vi "PS Control.vi"() -> ()   [LabVIEW 2023]
doc: "Author: Scott Hannahs <sth@magnet.fsu.edu>\nCopyright 2018 Florida State University, All rights reserved."
uses:
  SCM4 Interlock/RT SubVIs/RT System Auth Level.ctl
  SCM4 Interlock/RT SubVIs/PS Action Control.ctl
  <vilib>/Utility/miscctls.llb/LVOffsetAndMultiplierTypeDef.ctl
  SCM4 Interlock/RT SubVIs/Interlock RT FPGA Status Info.ctl
  SCM4 Interlock/FPGA SubVIs/FPGA Crowbar State.ctl
  SCM4 Interlock/RT SubVIs/Switch Box Status.ctl
  SubVIs/Interlock 32T Net Client Globals.vi
  TCP Functions/TCP Read Length and Value (STR).vi
  <vilib>/Utility/miscctls.llb/LVRectTypeDef.ctl
  <vilib>/Utility/miscctls.llb/LVPointTypeDef.ctl
panel:
  in  "Clear Quench":bool
  out "# Clients":u32
  out "Currents":dbl[][](graph)
  in  "Client Loop Time (mS)":u32=100
  out "Start DateStamp":timestamp format="%<%H:%M:%S%4u\n%Y/%m/%d>T"
  out "Version RT System":string
  out "Version FPGA":string
  in  "Password":string
  out "Authorized":T1
  in  "Slew Rate [T/min]":dbl format="%.3g"
  out "Field [T]":dbl format="%.5f"
  in  "Setpoint [T]":dbl format="%.6g"
  in  "PS Action":T2=enum."Hold"
  out "Version":string
  in  "stop":bool
  # "NHMFL 32T User Control"
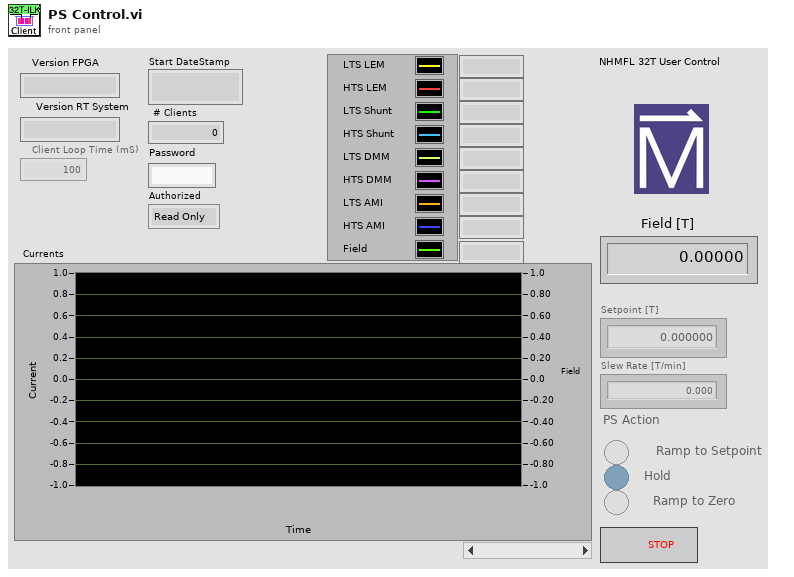
[diagram p1: front panel]
types:
  T1 = typedef "RT System Auth Level.ctl" = enum16{"Read Only", "User", "Operator", "Admin"}
  T2 = typedef "PS Action Control.ctl" = enum32{"Ramp to Setpoint", "Hold", "Ramp to Zero"}
  T3 = enum8{"Enabled", "Disabled", "Disabled and Grayed Out"}
  T4 = typedef "LVPointTypeDef.ctl" = cluster{"Horizontal":i16, "Vertical":i16}
  T5 = typedef "LVRectTypeDef.ctl" = cluster{"Left":i16, "Top":i16, "Right":i16, "Bottom":i16}
  T6 = typedef "LVOffsetAndMultiplierTypeDef.ctl" = cluster{"Offset":dbl, "Multiplier":dbl}
  T7 = enum16{"Standard", "Buffered", "CRLF", "Immediate"}
  T8 = typedef "Interlock RT FPGA Status Info.ctl" = cluster{"Authorized":T1, "# Clients":u32, "Chassis Temperature":fxp<+/-,16,14>, "Secondary QD Time Constant":enum16{"2000 mS", "1000 mS", "200 mS", "50 mS"}, "Crowbar Latch State":T9, "Crowbar Reset Countdown Length (ms)":i32, "Crowbar Reset Countdown":i32, "Ramp To Zero Fault":u32, "Crowbar Fault":u16, "Protection Logic V":dbl, "Quench Loop":dbl, "HTS LEM":dbl, "HTS Shunt":dbl, "LTS LEM":dbl, "LTS Shunt":dbl, "Ramp To Zero":bool, "2 Crowbar Reset Key":bool, "7 Crowbar LED":bool, "15 Close Switch Box 2 Contactor":bool, "HTS Voltage":dbl, "LTS Voltage":dbl, "DAQ Loop Ticks":u32, "PQD WDT Loop Tics":u32, "Main Loop Ticks":u32, "PS Check Loop Ticks":u32, "RTZ Loop Ticks":u32, "Watchdog Loop Ticks":u32, "LHe Level 1":dbl, "LHe Level 2":dbl, "HTS DMM":dbl, "LTS DMM":dbl, "HTS AMI430":dbl, "LTS AMI430":dbl, "Battery Monitor Alarm":bool, "Switch Box Status":T10, "PS Action":T2, "Setpoint [T]":dbl, "Field [T]":dbl, "Slew rate [T/min]":dbl, "Recorded error":errorcluster, "Last Batt Comm":timestamp, "Batt Alarm Text":string, "PS Comm Time (ms)":u32, "DMM Comm Time (ms)":u32, "PS Model Cluster":cluster{"HTS B_I0":dbl, "LTS B_I0":dbl, "HTS Bmax":dbl, "LTS Bmax":dbl, "Max combined rate (T/min)":dbl}, "HTS Setpoint [A]":dbl, "HTS Slew [A/S]":dbl, "LTS Setpoint [A]":dbl, "LTS Slew [A/S]":dbl}
  T9 = typedef "FPGA Crowbar State.ctl" = enum16{"Run", "Crowbar", "Reset Countdown"}
  T10 = typedef "Switch Box Status.ctl" = cluster{"Battery Voltage":dbl, "SwBox 1 Contactor V":dbl, "SwBox 2 Contactor V":dbl, "Battery Ground V":dbl}
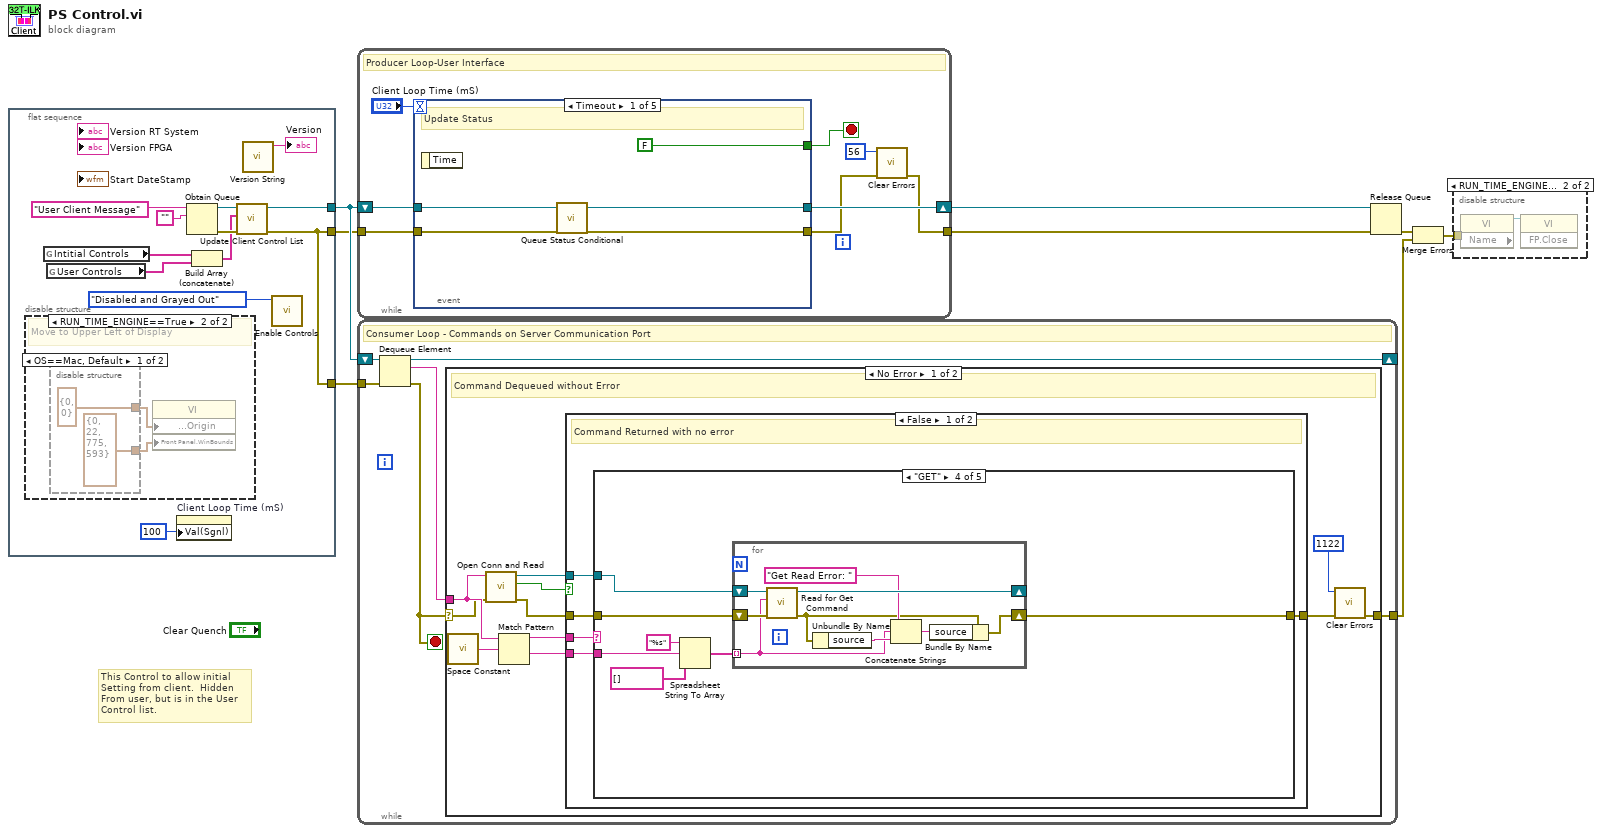
[diagram p0: block diagram]
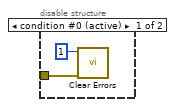
[diagram p2: hidden frame]
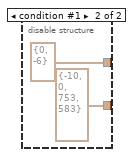
[diagram p4: hidden frame]
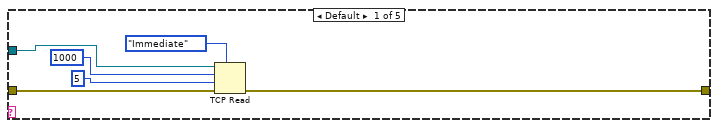
[diagram p5: hidden frame]
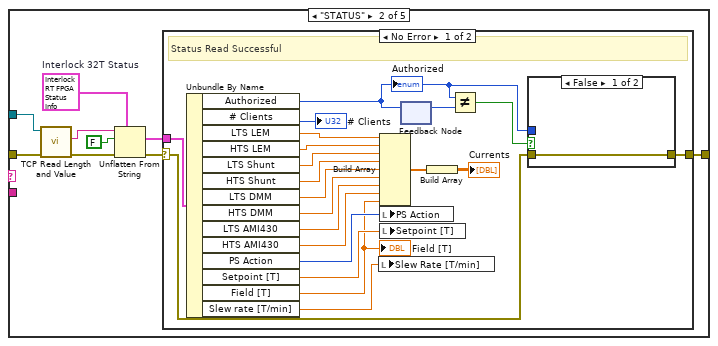
[diagram p6: hidden frame]
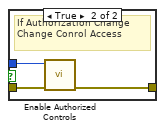
[diagram p7: hidden frame]
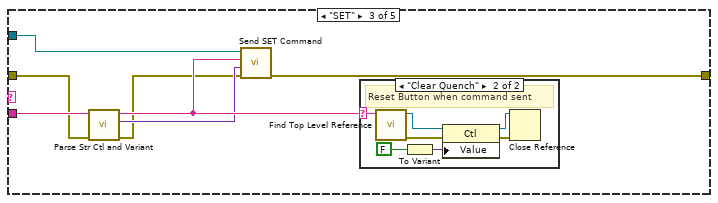
[diagram p9: hidden frame]
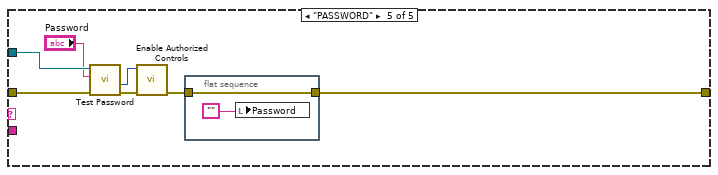
[diagram p11: hidden frame]
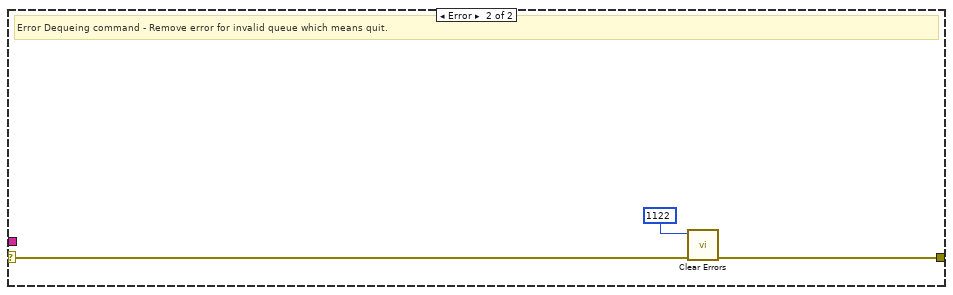
[diagram p13: hidden frame]
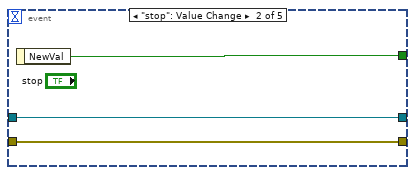
[diagram p14: hidden frame]
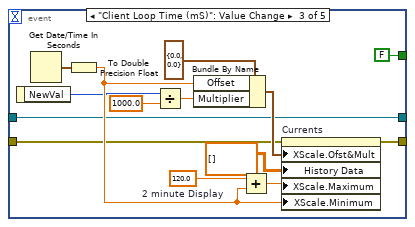
[diagram p15: hidden frame]
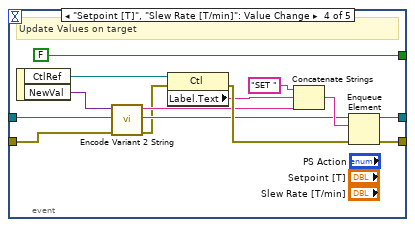
[diagram p16: hidden frame]
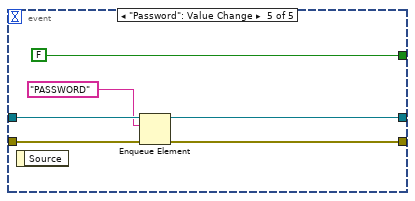
[diagram p17: hidden frame]
diagram:
  # "This Control to allow initial\nSetting from client.  Hidden\nFrom user, but is in the User\nControl list."
  n1 = flat-sequence {
    tunnel: [w20] -> w6
    tunnel: [w10] -> w3
    tunnel: [w10] -> w1
    frame #0 {
      n2 = disable-structure shown="RUN_TIME_ENGINE==True" {
        frame condition #0 (active) {
        }
        frame condition #1 {
          # "Move to Upper Left of Display"
          n3 = disable-structure shown="OS==Mac, Default" {
            disable-tunnel: [T5 {"Left"=0, "Top"=22, "Right"=775, "Bottom"=593} ("Front Panel Window:Window Bounds") T5 {"Left"=-10, "Top"=0, "Right"=753, "Bottom"=583} ("Front Panel Window:Window Bounds")] -> w22
            disable-tunnel: [T4 {"Horizontal"=0, "Vertical"=0} ("Front Panel Window:Origin") T4 {"Horizontal"=0, "Vertical"=-6} ("Front Panel Window:Origin")] -> w21
            frame condition #0 (active) {
            }
            frame condition #1 {
            }
          }
          n4 = property class="VI"("Front Panel Window:Origin"=w21, "Front Panel.WinBounds"=w22) -> ()  [unwired: 2 in, 2 out]
        }
      }
      n5 = global read "Interlock 32T Net Client Globals.vi" "Intitial Controls"() -> (w12:string[])
      n6 = global read "Interlock 32T Net Client Globals.vi" "User Controls"() -> (w11:string[])
      n7 = property on="Client Loop Time (mS)" class="DigNum (strict)"("Val(Sgnl)"=u32 100 ("Value (Signaling)")) -> ()  [unwired: 2 in, 2 out]
      n8 = Obtain Queue(name (unnamed)="User Client Message", element data type="") -> (queue out=w17:refnum<queue>, error out=w16:errorcluster)  [unwired: 3 in, 1 out]
      n9 = Build Array (concatenate)(w12, w11) -> (w14:string[])
      n10 = call "Update Client Control List.vi"("error in (no error)"=w16, "Array"=w14, "Queue in"=w17) -> ("error out"=w10:errorcluster, "Queue out"=w20:refnum<queue>)  [unwired: 6 in, 1 out]
      n11 = call "Version String.vi"() -> ("String"=→"Version":string)  [unwired: 10 in, 1 out]
      n12 = call "Enable Controls.vi"("Enable Disable"=T3."Disabled and Grayed Out") -> ()  [unwired: 10 in, 1 out]
    }
  }
  n13 = while {
    tunnel: w3 -> [w28]
    tunnel: [w29] -> w5
    shift-right: [w32] -> w8
    shift-left: w6 -> [w33]
    stop <- w30 stop-if-true
    # "Producer Loop-User Interface"
    n14 = event shown="[0] Timeout" {
      selector: _ -> [_ _ _ _ _]
      dyn-events: _ -> [_ _ _ _ _]
      timeout: "Client Loop Time (mS)" -> [_ _ _ _ _]
      tunnel: w28 -> [w38 w42 w43 w58 w74]
      tunnel: [w36 w42 w44 w63 w73] -> w31
      tunnel: [w35 w41 w46 w62 w72] -> w32
      tunnel: w33 -> [w37 w41 w46 w65 w75]
      tunnel: [FALSE ("NewVal") w40 FALSE ("NewVal") FALSE ("NewVal") FALSE ("NewVal")] -> w30
      event Timeout {
        # "Update Status"
        n15 = event-data() -> ()  [unwired: 1 in, 1 out]
        n16 = call "Queue Status Conditional.vi"("error in (no error)"=w38, "Queue in"=w37) -> ("error out"=w36:errorcluster, "Queue out"=w35:refnum<queue>)  [unwired: 8 in]
      }
      event "stop": Value Change {
        n17 = event-data() -> ("NewVal"=w40:bool)  [unwired: 1 in]
      }
      event "Client Loop Time (mS)": Value Change {
        w51 = 120.0  # 2 minute Display
        n18 = event-data() -> ("NewVal"=w47:u32)  [unwired: 1 in]
        n19 = Get Date/Time In Seconds() -> (seconds since 1Jan1904=w52:timestamp)
        n20 = To Double Precision Float(number=w52) -> (double precision float=w56:dbl)
        n21 = Divide(x=w47, y=1000.0) -> (x/y=w54:dbl)
        n22 = Bundle By Name(cluster=T6 {"Offset"=0.0, "Multiplier"=0.0} ("X Scale.Offset and Multiplier"), "Offset"=w56, "Multiplier"=w54) -> (w53:T6)
        n23 = Add(x=w51, y=w56) -> (x+y=w55:dbl)
        n24 = property on="Currents" class="WFChart (strict)"(error in=w43, "XScale.Ofst&Mult"=w53, "History Data"=dbl[][] [], "XScale.Maximum"=w55, "XScale.Minimum"=w56) -> (error out=w44:errorcluster)  [unwired: 1 in, 1 out]
      }
      event "Setpoint [T]", "Slew Rate [T/min]": Value Change {
        # "Update Values on target"
        n25 = event-data() -> ("CtlRef"=w69:refnum<vi>, "NewVal"=w59:variant)  [unwired: 1 in]
        n26 = call "Encode Variant 2 String.vi"("error in"=w58, "Variant"=w59) -> ("error out"=w57:errorcluster, "String Output"=w60:string)  [unwired: 8 in]
        n27 = property class="Ctl"(reference=w69, error in=w57) -> (error out=w67:errorcluster, "Label.Text"=w64:string)  [unwired: 1 out]
        n28 = Concatenate Strings("SET " ("string"), w64, w60) -> (w66:string)
        n29 = Enqueue Element(queue=w65, element=w66, error in (no error)=w67) -> (queue out=w62:refnum<queue>, error out=w63:errorcluster)  [unwired: 1 in, 1 out]
      }
      event "Password": Value Change {
        n30 = event-data() -> ()  [unwired: 1 in, 1 out]
        n31 = Enqueue Element(queue=w75, element="PASSWORD" ("string"), error in (no error)=w74) -> (queue out=w72:refnum<queue>, error out=w73:errorcluster)  [unwired: 1 in, 1 out]
      }
    }
    n32 = call <vilib>:"Clear Errors.vi"("error in (no error)"=w31, "specific error code to clear (0: all)"=56) -> ("error out"=w29:errorcluster)  [unwired: 4 in, 1 out]
  }
  n33 = while {
    shift-right: [w79] -> _
    shift-left: w6 -> [w81]
    tunnel: w1 -> [w80]
    tunnel: [w76] -> w4
    stop <- w77 stop-if-true
    # "Consumer Loop - Commands on Server Communication Port"
    n34 = Dequeue Element(queue=w81, error in (no error)=w80) -> (queue out=w79:refnum<queue>, element=w78:string, error out=w77:errorcluster)  [unwired: 1 in, 1 out]
    n35 = case shown="No Error" w77 {
      selector: w77 -> [w85 w181]
      tunnel: [w83 w180] -> w76
      tunnel: w78 -> [w89 _]
      frame No Error {
        # "Command Dequeued without Error"
        n36 = call <vilib>:"Space Constant.vi"() -> ("String"=w87:string)
        n37 = call "Open Conn and Read.vi"("error in (no error)"=w85, "String"=w89) -> ("error out"=w91:errorcluster, "Returned Error"=w90:bool, "TCP Network Connection out"=w92:refnum<k5>)  [unwired: 6 in, 1 out]
        n38 = Match Pattern(string=w89, regular expression=w87) -> (before substring=w88:string, after substring=w86:string)  [unwired: 1 in, 2 out]
        n39 = case shown="False" w90 {
          tunnel: [w97 w178] -> w82
          tunnel: w92 -> [w96 _]
          tunnel: w91 -> [w95 w178]
          tunnel: w88 -> [w94 _]
          tunnel: w86 -> [w93 _]
          frame False {
            # "Command Returned with no error"
            n40 = case shown="\"GET\"" w94 {
              tunnel: [w98 w104 w145 w153 w172] -> w97
              tunnel: w95 -> [w100 w111 w140 w159 w175]
              tunnel: w96 -> [w99 w110 w144 w155 w174]
              tunnel: w93 -> [_ _ w143 w154 _]
              frame Default {
                n41 = TCP Read(connection ID=w99, bytes to read=1000, error in (no error)=w100, 7:T7."Immediate" ("mode (standard)"), 9:5 ("timeout ms (25000)")) -> (error out=w98:errorcluster)  [unwired: 2 out]
              }
              frame "STATUS" {
                w106 = T8 {"Authorized"=enum."Read Only", "# Clients"=0, "Chassis Temperature"=0.0, "Secondary QD Time Constant"=enum."2000 mS", "Crowbar Latch State"=enum."Run", "Crowbar Reset Countdown Length (ms)"=0, "Crowbar Reset Countdown"=0, "Ramp To Zero Fault"=0, "Crowbar Fault"=0, "Protection Logic V"=0.0, "Quench Loop"=0.0, "HTS LEM"=0.0, "HTS Shunt"=0.0, "LTS LEM"=0.0, "LTS Shunt"=0.0, "Ramp To Zero"=FALSE, "2 Crowbar Reset Key"=FALSE, "7 Crowbar LED"=FALSE, "15 Close Switch Box 2 Contactor"=FALSE, "HTS Voltage"=0.0, "LTS Voltage"=0.0, "DAQ Loop Ticks"=0, "PQD WDT Loop Tics"=0, "Main Loop Ticks"=0, "PS Check Loop Ticks"=0, "RTZ Loop Ticks"=0, "Watchdog Loop Ticks"=0, "LHe Level 1"=2.148782730102539, "LHe Level 2"=3.334085464477539, "HTS DMM"=0.0, "LTS DMM"=0.0, "HTS AMI430"=0.0, "LTS AMI430"=0.0, "Battery Monitor Alarm"=FALSE, "Switch Box Status"={"Battery Voltage"=0.0, "SwBox 1 Contactor V"=0.0, "SwBox 2 Contactor V"=0.0, "Battery Ground V"=0.0}, "PS Action"=enum."Ramp to Zero", "Setpoint [T]"=0.0, "Field [T]"=0.0, "Slew rate [T/min]"=0.01, "Recorded error"={"status"=FALSE, "code"=0, "source"=""}, "Last Batt Comm"=timestamp(0 s since 1904-01-01), "Batt Alarm Text"="", "PS Comm Time (ms)"=0, "DMM Comm Time (ms)"=0, "PS Model Cluster"={"HTS B_I0"=0.0, "LTS B_I0"=0.0, "HTS Bmax"=0.0, "LTS Bmax"=0.0, "Max combined rate (T/min)"=0.0}, "HTS Setpoint [A]"=0.0, "HTS Slew [A/S]"=0.0, "LTS Setpoint [A]"=0.0, "LTS Slew [A/S]"=0.0}  # Interlock 32T Status
                n42 = call-poly "TCP Read Length and Value.vi"("error in (no error)"=w111, "TCP Network Connection in"=w110) -> ("error out"=w112:errorcluster, "Output"=w108:string)  [unwired: 7 in, 1 out]
                n43 = Unflatten From String(type=w106, binary string=w108, data includes array or string size? (T)=FALSE, error in (no error)=w112) -> (value=w109:T8, error out=w105:errorcluster)  [unwired: 1 in, 1 out]
                n44 = case shown="No Error" w105 {
                  selector: w105 -> [w129 w138]
                  tunnel: w109 -> [w133 _]
                  tunnel: [w128 w138] -> w104
                  frame No Error {
                    # "Status Read Successful"
                    n45 = Unbundle By Name(w133) -> ("Authorized"=w130:T1, "# Clients"=→"# Clients":u32, "LTS LEM"=w125:dbl, "HTS LEM"=w124:dbl, "LTS Shunt"=w122:dbl, "HTS Shunt"=w121:dbl, "LTS DMM"=w117:dbl, "HTS DMM"=w116:dbl, "LTS AMI430"=w115:dbl, "HTS AMI430"=w114:dbl, "PS Action"=w120:T2, "Setpoint [T]"=w119:dbl, "Field [T]"=w113:dbl, "Slew rate [T/min]"=w118:dbl)
                    "Authorized" <- w130
                    "Field [T]" <- w113
                    n46 = local write "Slew Rate [T/min]"(w118) -> ()
                    n47 = Build Array(w125, w124, w122, w121, w117, w116, w115, w114, w113) -> (w127:dbl[])
                    n48 = local write "PS Action"(w120) -> ()
                    n49 = local write "Setpoint [T]"(w119) -> ()
                    n50 = feedback-in #1(w130) -> ()
                    n51 = feedback #1() -> (w132:T1)  [unwired: 1 in]
                    n52 = Build Array(w127) -> (→"Currents":dbl[][])
                    n53 = Not Equal?(x=w130, y=w132) -> (x != y?=w131:bool)
                    n54 = case shown="False" w131 {
                      tunnel: w130 -> [_ w137]
                      tunnel: w129 -> [w134 w136]
                      tunnel: [w134 w135] -> w128
                      frame False {
                      }
                      frame True {
                        # "If Authorization Change\nChange Conrol Access"
                        n55 = call "Enable Authorized Controls.vi"("error in (no error)"=w136, "Authorized"=w137) -> ("error out"=w135:errorcluster)  [unwired: 9 in]
                      }
                    }
                  }
                  frame Error {
                    # "Status Not Read"
                  }
                }
              }
              frame "SET" {
                n56 = call "Parse Str Ctl and Variant.vi"("error in"=w140, "String Input"=w143) -> ("error out"=w139:errorcluster, "variant output"=w141:variant, "Control Name"=w142:string)  [unwired: 7 in]
                n57 = call "Send SET Command.vi"("error in (no error)"=w139, "Control Value"=w141, "Control Name"=w142, "TCP Network Connection in"=w144) -> ("error out"=w145:errorcluster)  [unwired: 7 in]
                n58 = case shown="\"Clear Quench\"" w142 {
                  selector: w142 -> [_ w152]
                  frame Default {
                  }
                  frame "Clear Quench" {
                    # "Reset Button when command sent"
                    n59 = call "Find Top Level Reference.vi"("String"=w152) -> ("error out"=w147:errorcluster, "Ctl Refnum"=w151:refnum<vi>)  [unwired: 9 in]
                    n60 = To Variant(anything=FALSE) -> (Variant=w146:variant)
                    n61 = property class="Ctl"(reference=w151, error in=w147, "Value"=w146) -> (reference out=w148:refnum<vi>, error out=w149:errorcluster)
                    n62 = Close Reference(reference=w148, error in (no error)=w149) -> ()  [unwired: 1 out]
                  }
                }
              }
              frame "GET" {
                n63 = Spreadsheet String To Array(format string="%s", spreadsheet string=w154, array type (2D Dbl)=string[] []) -> (array=w158:string[])  [unwired: 1 in]
                n64 = for {
                  tunnel: w158 -> [w160] mode=indexing
                  shift-right: [w162] -> w153
                  shift-left: w159 -> [w167]
                  shift-right: [w166] -> _
                  shift-left: w155 -> [w168]
                  n65 = call "Read for Get Command.vi"("error in (no error)"=w167, "Control Name"=w160, "TCP Network Connection in"=w168) -> ("error out"=w161:errorcluster, "TCP Network Connection out"=w166:refnum<k5>)  [unwired: 7 in]
                  n66 = Unbundle By Name(w161) -> ("source"=w164:string)
                  n67 = Concatenate Strings("Get Read Error: " ("string"), w160, w164) -> (w165:string)
                  n68 = Bundle By Name(cluster=w161, "source"=w165) -> (w162:errorcluster)
                }
              }
              frame "PASSWORD" {
                n69 = call "Test Password.vi"("error in (no error)"=w175, "String"="Password", "TCP Network Connection in"=w174) -> ("error out"=w169:errorcluster, "Authorized"=w171:T1)  [unwired: 6 in, 1 out]
                n70 = call "Enable Authorized Controls.vi"("error in (no error)"=w169, "Authorized"=w171) -> ("error out"=w170:errorcluster)  [unwired: 9 in]
                n71 = flat-sequence {
                  tunnel: w170 -> [w177]
                  tunnel: [w177] -> w172
                  frame #0 {
                    n72 = local write "Password"("") -> ()
                  }
                }
              }
            }
          }
          frame True {
          }
        }
        n73 = call <vilib>:"Clear Errors.vi"("error in (no error)"=w82, "specific error code to clear (0: all)"=1122) -> ("error out"=w83:errorcluster)  [unwired: 4 in, 1 out]
      }
      frame Error {
        # "Error Dequeing command - Remove error for invalid queue which means quit."
        n74 = call <vilib>:"Clear Errors.vi"("error in (no error)"=w181, "specific error code to clear (0: all)"=1122) -> ("error out"=w180:errorcluster)  [unwired: 4 in, 1 out]
      }
    }
  }
  n75 = Release Queue(queue=w8, error in (no error)=w5) -> (error out=w7:errorcluster)  [unwired: 1 in, 2 out]
  n76 = Merge Errors(w7, w4) -> (w2:errorcluster)
  n77 = disable-structure shown="RUN_TIME_ENGINE==True" {
    disable-tunnel: w2 -> [w183 _]
    frame condition #0 (active) {
      n78 = call <vilib>:"Clear Errors.vi"("error in (no error)"=w183, "specific error code to clear (0: all)"=1) -> ()  [unwired: 4 in, 2 out]
    }
    frame condition #1 {
      n79 = property class="VI" props=["Name"]() -> (reference out=w184:refnum<vi>)  [unwired: 2 in, 2 out]
      n80 = invoke class="VI" method="FP.Close"(reference=w184) -> ()  [unwired: 2 in, 3 out]
    }
  }
